vi "Apply Optical PWM To Enable.vi"(0 "Pulse Train in":refnum<class "Pulse Train.lvclass">, 7 "Pulse width (us)":dbl, 9 "PWM factor":dbl, 11 "error in (no error)":errorcluster) -> (4 "Pulse Train out":refnum<class "Pulse Train.lvclass">, 15 "error out":errorcluster)   [LabVIEW 2015, in "Pulse Train.lvclass"]
uses:
  Pulse Train.lvclass
  Pulse Train.lvclass/Pulse Train.ctl
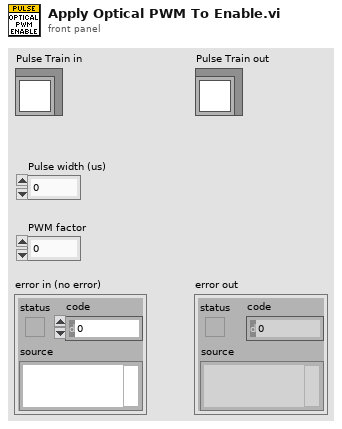
[diagram p1: front panel]
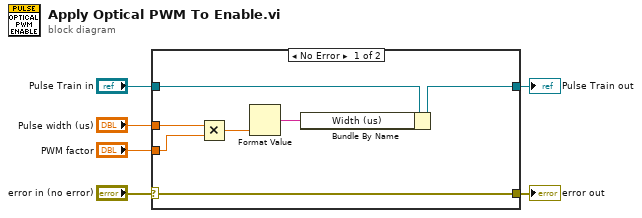
[diagram p0: block diagram]
diagram:
  n1 = case shown="No Error" "error in (no error)" {
    selector: "error in (no error)" -> [w13 w15]
    tunnel: [w13 w15] -> w5
    tunnel: [w9 w14] -> w3
    tunnel: "Pulse Train in" -> [w12 w14]
    tunnel: "PWM factor" -> [w10 _]
    tunnel: "Pulse width (us)" -> [w11 _]
    frame No Error {
      n2 = Multiply(x=w11, y=w10) -> (x*y=w8:dbl)
      n3 = Format Value(value (0)=w8) -> (output string=w7:string)  [unwired: 2 in]
      n4 = Bundle By Name(cluster=w12, "Width (us)"=w7) -> (w9:refnum<class "Pulse Train.lvclass">)
    }
    frame Error {
    }
  }
  "error out" <- w5
  "Pulse Train out" <- w3
